vi "Set End Time.vi"(11 "Test Suite In":refnum<class "LUnit Test Suite.lvclass">) -> (3 "Test Suite Out":refnum<class "LUnit Test Suite.lvclass">)   [LabVIEW 2020, in "LUnit Test Suite.lvclass"]
doc: "Generate test suite results."
uses:
  LUnit Test Suite.lvclass
  LUnit Test Suite.lvclass/LUnit Test Suite.ctl
  Result Classes/Test Suite Result/Test Suite Result.lvclass/Test Suite Result.ctl
  Result Classes/Test Suite Result/Test Suite Result.lvclass
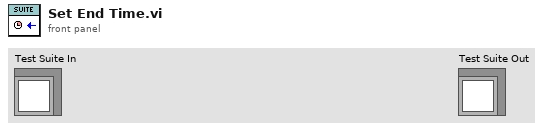
[diagram p1: front panel]
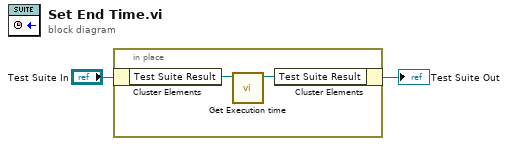
[diagram p0: block diagram]
diagram:
  n1 = in-place {
    n2 = in-place-cluster #1("Test Suite In") -> ("Test Suite Result"=w4:refnum<class "Test Suite Result.lvclass">)
    n3 = call "Get Execution time.vi"("Test Suite Result In"=w4) -> ("Test Suite Result Out"=w3:refnum<class "Test Suite Result.lvclass">)  [unwired: 10 in]
    n4 = in-place-cluster #1("Test Suite Result"=w3) -> (→"Test Suite Out":refnum<class "LUnit Test Suite.lvclass">)
  }
